vi "LoggerManager.vi"   [LabVIEW 2014]
uses:
  <vilib>/Rock Robotics/WPI/RobotDrive/WPI_RobotDriveGetSetRefNum.vi
  <vilib>/Rock Robotics/WPI/Solenoid/WPI_SolenoidGetEnum.vi
  <vilib>/Rock Robotics/Network Tables/SD Write String.vi
types:
  T1 = typedef "WPI_RobotDriveDevRef.ctl" = cluster{"DevStatus":errorcluster, "Motors[]":T2[], "Square Inputs":bool, "Max Output":dbl}
  T2 = typedef "WPI_MotorControlDeviceRef.ctl" = cluster{"DeviceStatus":errorcluster, "Type":T3, "PWM":cluster{"Controller":T4, "PWM Channel":T5, "DeadBand":T6}, "CAN":cluster{"Device Number":u8, "Control Mode":T7, "Semaphore":T8, "Max Vout":dbl, "TalonSRX Control Mode":T9}, "Invert":bool, "TransformRef":T10, "InvTransformRef":T10}
  T3 = typedef "WPI_MotorControlType.ctl" = enum16{"PWM", "CAN", "CANTalonSRX"}
  T4 = typedef "FPGA_TypedefDigitalModule.ctl" = enum16{"Controller 1"}
  T5 = typedef "FPGA_DIOPWMChannel.ctl" = enum8{"PWM 0", "PWM 1", "PWM 2", "PWM 3", "PWM 4", "PWM 5", "PWM 6", "PWM 7", "PWM 8", "PWM 9", "PWM MXP 0", "PWM MXP 1", "PWM MXP 2", "PWM MXP 3", "PWM MXP 4", "PWM MXP 5", "PWM MXP 6", "PWM MXP 7", "PWM MXP 8", "PWM MXP 9", "Invalid"}
  T6 = typedef "WPI_PWMDeadband.ctl" = cluster{"Name":string, "maxPositivePwm":i32, "minPositivePwm":i32, "centerPwm":i32, "maxNegativePwm":i32, "minNegativePwm":i32, "angularRange":u16}
  T7 = typedef "WPI_CANJaguar_ControlMode.ctl" = enum8{"Percent VBus", "Current", "Speed", "Position", "Voltage"}
  T8 = typedef "Semaphore RefNum" = refnum<k1>
  T9 = typedef "WPI_CANTalonSRX_APIControlMode.ctl" = enum8{"Percent VBus", "Speed", "Position", "Slave", "Unchanged / Invalid"}
  T10 = typedef "WPI_PWMTransform_ConPane.ctl" = refnum<vi>
  T11 = typedef "WPI_CANTalonSRX_GlobalStatus.ctl" = cluster{"Applied Throttle":dbl, "Module Enabled":bool, "CAN Error":errorcluster, "Closed Loop Error":dbl, "Forward Limit Switch Closed":bool, "Reverse Limit Switch Closed":bool, "Sensor Position":dbl, "Sensor Velocity":dbl, "Current":dbl, "Sticky Fault - Over Temp":bool, "Sticky Fault - Under Voltage":bool, "Sticky Fault - Forward Limit":bool, "Sticky Fault - Reverse Limit":bool, "Sticky Fault - Forward Soft Limit":bool, "Sticky Fault - Reverse Soft Limit":bool, "Brake is Enabled":bool, "Encoder Position":dbl, "Encoder Velocity":dbl, "Encoder Index Count":dbl, "Encoder A Pin State":bool, "Encoder B Pin State":bool, "Encoder Index Pin State":bool, "Analog In":dbl, "Analog In Velocity":dbl, "Temperature (C)":dbl, "Battery Voltage":dbl}
  T12 = typedef "WPI_SolenoidDevRef.ctl" = cluster{"DevStatus":errorcluster, "Pneumatics Control Module":u8, "Forward Solenoid Channel":T13, "Reverse Solenoid Channel":T13}
  T13 = typedef "WPI_SolenoidChannel.ctl" = enum8{"Solenoid 0", "Solenoid 1", "Solenoid 2", "Solenoid 3", "Solenoid 4", "Solenoid 5", "Solenoid 6", "Solenoid 7", "Invalid"}
  T14 = typedef "WPI_SolenoidValue.ctl" = enum16{"Off", "On", "Forward", "Reverse"}
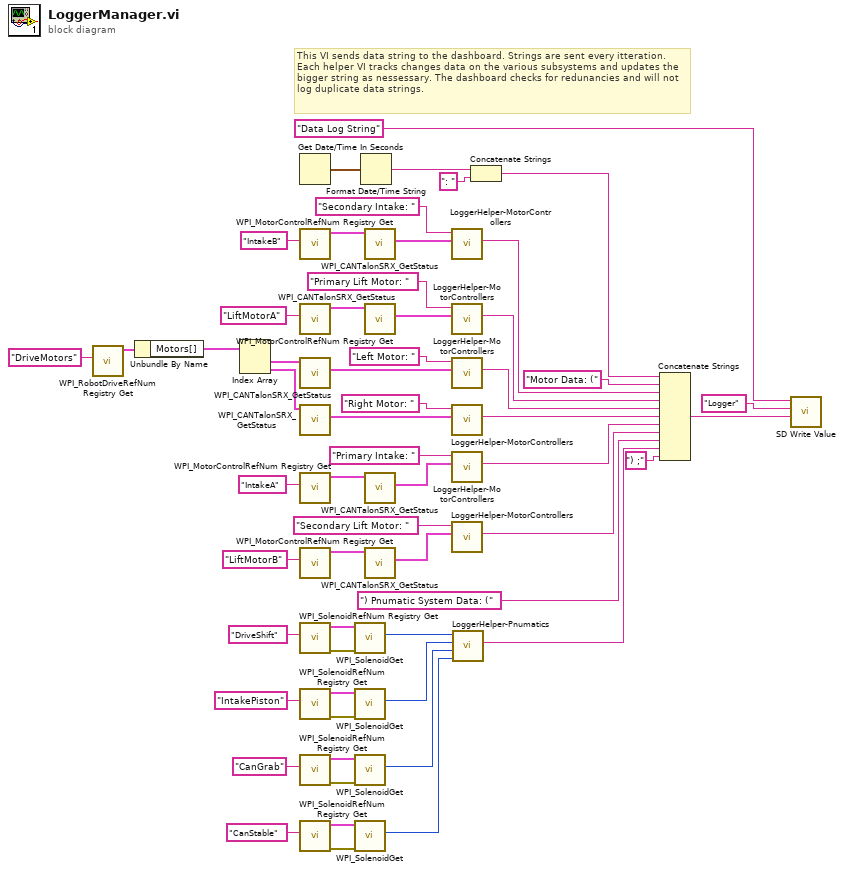
[diagram p0: block diagram]
diagram:
  # "This VI sends data string to the dashboard. Strings are sent every itteration. Each helper VI tracks changes data on the various subsystems and updates the bigger string as nessessary. The dashboard checks for redunancies and will not log duplicate data strings."
  n1 = call <vilib>:"WPI_RobotDriveRefNum Registry Get.vi"("refnum name"="DriveMotors") -> ("RobotDriveDevRef"=w53:T1)  [unwired: 9 in, 1 out]
  n2 = Unbundle By Name(w53) -> ("Motors[]"=w52:T2[])
  n3 = Index Array(array=w52) -> (element #1=w51:T2, element #2=w50:T2)  [unwired: 2 in]
  n4 = Get Date/Time In Seconds() -> (seconds since 1Jan1904=w45:timestamp)
  n5 = call <vilib>:"WPI_MotorControlRefNum Registry Get.vi"("refnum name"="IntakeB") -> ("MotorControlDevRef"=w48:T2)  [unwired: 9 in, 1 out]
  n6 = call <vilib>:"WPI_MotorControlRefNum Registry Get.vi"("refnum name"="LiftMotorA") -> ("MotorControlDevRef"=w47:T2)  [unwired: 9 in, 1 out]
  n7 = call <vilib>:"WPI_CANTalonSRX_GetStatus.vi"("CAN Talon SRX Ref"=w51) -> ("Talon SRX Status"=w32:T11)  [unwired: 8 in, 2 out]
  n8 = call <vilib>:"WPI_CANTalonSRX_GetStatus.vi"("CAN Talon SRX Ref"=w50) -> ("Talon SRX Status"=w33:T11)  [unwired: 8 in, 2 out]
  n9 = call <vilib>:"WPI_MotorControlRefNum Registry Get.vi"("refnum name"="IntakeA") -> ("MotorControlDevRef"=w49:T2)  [unwired: 9 in, 1 out]
  n10 = call <vilib>:"WPI_MotorControlRefNum Registry Get.vi"("refnum name"="LiftMotorB") -> ("MotorControlDevRef"=w46:T2)  [unwired: 9 in, 1 out]
  n11 = call <vilib>:"WPI_SolenoidRefNum Registry Get.vi"("refnum name"="DriveShift") -> ("error out"=w17:errorcluster, "SolenoidDevRef"=w16:T12)  [unwired: 9 in]
  n12 = call <vilib>:"WPI_SolenoidRefNum Registry Get.vi"("refnum name"="IntakePiston") -> ("error out"=w19:errorcluster, "SolenoidDevRef"=w18:T12)  [unwired: 9 in]
  n13 = call <vilib>:"WPI_SolenoidRefNum Registry Get.vi"("refnum name"="CanGrab") -> ("error out"=w4:errorcluster, "SolenoidDevRef"=w3:T12)  [unwired: 9 in]
  n14 = call <vilib>:"WPI_SolenoidRefNum Registry Get.vi"("refnum name"="CanStable") -> ("error out"=w6:errorcluster, "SolenoidDevRef"=w5:T12)  [unwired: 9 in]
  n15 = call-poly <vilib>:"WPI_SolenoidGet.vi"("error in (no error)"=w17, "SolenoidDevRef"=w16) -> ("Value"=w11:T14)  [unwired: 7 in, 2 out]
  n16 = call-poly <vilib>:"WPI_SolenoidGet.vi"("error in (no error)"=w19, "SolenoidDevRef"=w18) -> ("Value"=w10:T14)  [unwired: 7 in, 2 out]
  n17 = call-poly <vilib>:"WPI_SolenoidGet.vi"("error in (no error)"=w4, "SolenoidDevRef"=w3) -> ("Value"=w2:T14)  [unwired: 7 in, 2 out]
  n18 = call-poly <vilib>:"WPI_SolenoidGet.vi"("error in (no error)"=w6, "SolenoidDevRef"=w5) -> ("Value"=w1:T14)  [unwired: 7 in, 2 out]
  n19 = Format Date/Time String(seconds (now)=w45) -> (date/time string=w44:string)  [unwired: 2 in]
  n20 = call <vilib>:"WPI_CANTalonSRX_GetStatus.vi"("CAN Talon SRX Ref"=w48) -> ("Talon SRX Status"=w35:T11)  [unwired: 8 in, 2 out]
  n21 = call <vilib>:"WPI_CANTalonSRX_GetStatus.vi"("CAN Talon SRX Ref"=w47) -> ("Talon SRX Status"=w40:T11)  [unwired: 8 in, 2 out]
  n22 = call <vilib>:"WPI_CANTalonSRX_GetStatus.vi"("CAN Talon SRX Ref"=w49) -> ("Talon SRX Status"=w34:T11)  [unwired: 8 in, 2 out]
  n23 = call <vilib>:"WPI_CANTalonSRX_GetStatus.vi"("CAN Talon SRX Ref"=w46) -> ("Talon SRX Status"=w43:T11)  [unwired: 8 in, 2 out]
  n24 = call "LoggerHelper-MotorControllers.vi"("Talon SRX Status Input"=w35, "Prefix Name"="Secondary Intake: ") -> ("Talon Log Data"=w26:string)  [unwired: 9 in]
  n25 = call "LoggerHelper-MotorControllers.vi"("Talon SRX Status Input"=w40, "Prefix Name"="Primary Lift Motor: ") -> ("Talon Log Data"=w27:string)  [unwired: 9 in]
  n26 = call "LoggerHelper-MotorControllers.vi"("Talon SRX Status Input"=w32, "Prefix Name"="Left Motor: ") -> ("Talon Log Data"=w28:string)  [unwired: 9 in]
  n27 = call "LoggerHelper-MotorControllers.vi"("Talon SRX Status Input"=w33, "Prefix Name"="Right Motor: ") -> ("Talon Log Data"=w29:string)  [unwired: 9 in]
  n28 = call "LoggerHelper-MotorControllers.vi"("Talon SRX Status Input"=w34, "Prefix Name"="Primary Intake: ") -> ("Talon Log Data"=w30:string)  [unwired: 9 in]
  n29 = call "LoggerHelper-MotorControllers.vi"("Talon SRX Status Input"=w43, "Prefix Name"="Secondary Lift Motor: ") -> ("Talon Log Data"=w31:string)  [unwired: 9 in]
  n30 = call "LoggerHelper-Pnumatics.vi"("Stablizer"=w1, "Grabber"=w2, "Intake"=w10, "Shifter"=w11) -> ("Logged PNU Output"=w9:string)  [unwired: 7 in]
  n31 = Concatenate Strings(w44, ": " ("string")) -> (w15:string)
  n32 = Concatenate Strings(w15, "Motor Data: (" ("Name"), w26, w27, w28, w29, w30, w31, ") Pnumatic System Data: (" ("string"), w9, ") ;" ("string")) -> (w24:string)
  n33 = call-poly <vilib>:"SD Write Value.vi"("String"=w24, "Table Prefix"="Logger", "Name"="Data Log String") -> ()  [unwired: 7 in, 2 out]
